vi "CheckSum.vi"(1 "Input String Array":string[](array[string])) -> (0 "Output String Array":string[](array[string]))   [LabVIEW 2014]
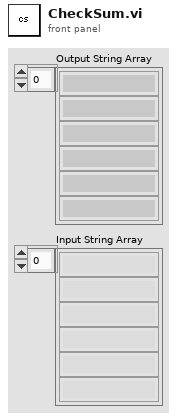
[diagram p1: front panel]
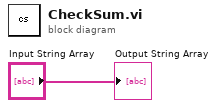
[diagram p0: block diagram]
diagram:
  "Output String Array" <- "Input String Array"
